vi "Display.vi"(8 "error in":errorcluster, 10 "Sub Panel":refnum<vi>, 11 "Configurator Actor:Configuration UI Actor in":refnum<class "Configuration UI Actor.lvclass">) -> (0 "error out":errorcluster, 3 "Configurator Actor:Configuration UI Actor out":refnum<class "Configuration UI Actor.lvclass">)   [LabVIEW 2023, in "Configuration UI Actor.lvlib" / "Configuration UI Actor.lvclass"]
uses:
  Configuration UI Actor.lvclass
  Configuration UI Actor.lvclass/Configuration UI Actor.ctl
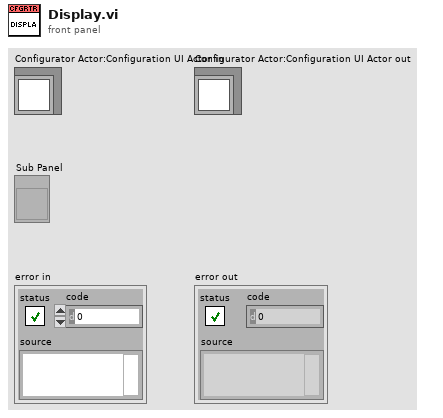
[diagram p1: front panel]
types:
  T1 = enum32{"Invalid", "Standard", "Closed", "Hidden", "Minimized", "Maximized"}
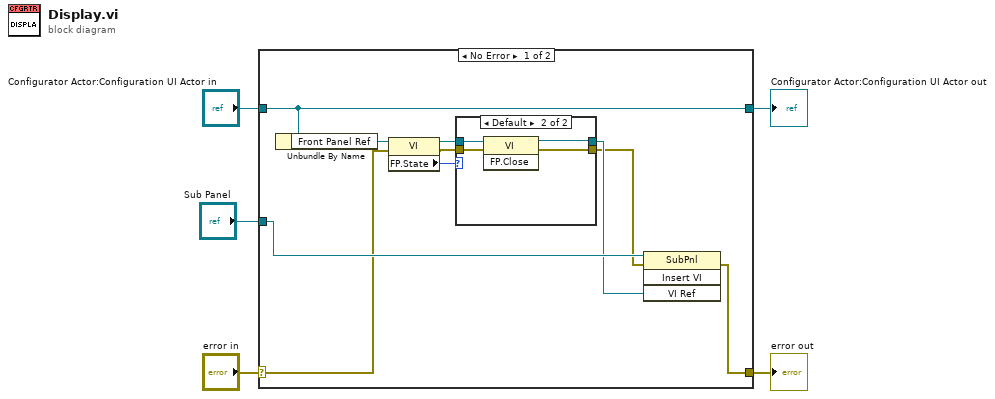
[diagram p0: block diagram]
diagram:
  n1 = case shown="No Error" "error in" {
    selector: "error in" -> [w7 w23]
    tunnel: [w6 w23] -> w4
    tunnel: [w15 w22] -> w2
    tunnel: "Configurator Actor:Configuration UI Actor in" -> [w15 w22]
    tunnel: "Sub Panel" -> [w11 _]
    frame No Error {
      n2 = Unbundle By Name(w15) -> ("Front Panel Ref"=w14:refnum<vi>)
      n3 = property class="VI"(reference=w14, error in=w7) -> (reference out=w12:refnum<vi>, error out=w8:errorcluster, "FP.State"=w13:T1)
      n4 = case shown="Default" w13 {
        tunnel: w12 -> [w17 w20]
        tunnel: [w17 w19] -> w10
        tunnel: [w16 w18] -> w9
        tunnel: w8 -> [w16 w21]
        frame "Closed" {
        }
        frame Default {
          n5 = invoke class="VI" method="FP.Close"(reference=w20, error in=w21) -> (reference out=w19:refnum<vi>, error out=w18:errorcluster)  [unwired: 1 in, 1 out]
        }
      }
      n6 = invoke class="SubPnl" method="Insert VI"(reference=w11, error in=w9, "VI Ref"=w10) -> (error out=w6:errorcluster)  [unwired: 1 in, 3 out]
    }
    frame Error {
    }
  }
  "error out" <- w4
  "Configurator Actor:Configuration UI Actor out" <- w2
